vi "test_libssh2_channel_get_exit_signal.vi"() -> ()   [LabVIEW 2017, in "integration_tests.lvlib"]
uses:
  integration_tests.lvlib
  libssh2/libssh2_channel_open_ex.vi
  libssh2/libssh2_channel_process_startup.vi
  support/support.lvlib
  libssh2/libssh2.lvlib
  <vilib>/PNR/Transparent Assertions/Transparent Assertions/Transparent Assertions.lvlib
panel:
  out "error out":errorcluster
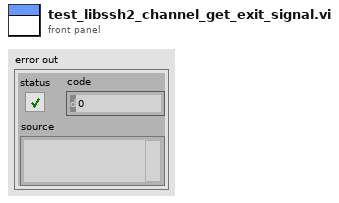
[diagram p1: front panel]
types:
  T1 = typedef "libssh2.lvlib/Session Refnum.ctl" = refnum<k1>
  T2 = typedef "libssh2.lvlib/Channel Refnum.ctl" = refnum<k1>
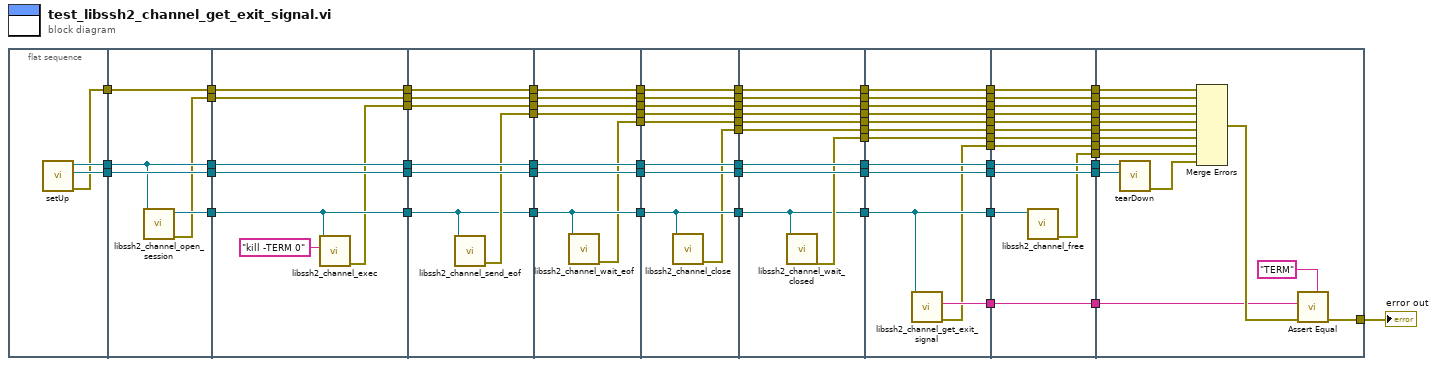
[diagram p0: block diagram]
diagram:
  n1 = flat-sequence {
    tunnel: [w76] -> w73
    tunnel: [w75] -> w72
    tunnel: [w74] -> w71
    tunnel: w73 -> [w80]
    tunnel: w72 -> [w81]
    tunnel: [w80] -> w70
    tunnel: [w81] -> w69
    tunnel: [w79] -> w68
    tunnel: w71 -> [w78]
    tunnel: [w78] -> w67
    tunnel: [w77] -> w66
    tunnel: w70 -> [w88]
    tunnel: [w88] -> w65
    tunnel: w69 -> [w87]
    tunnel: [w87] -> w64
    tunnel: w68 -> [w84]
    tunnel: [w84] -> w63
    tunnel: w67 -> [w86]
    tunnel: [w86] -> w62
    tunnel: w66 -> [w83]
    tunnel: [w83] -> w61
    tunnel: [w82] -> w60
    tunnel: w65 -> [w95]
    tunnel: [w95] -> w19
    tunnel: w64 -> [w94]
    tunnel: [w94] -> w17
    tunnel: w63 -> [w89]
    tunnel: [w89] -> w15
    tunnel: w62 -> [w93]
    tunnel: [w93] -> w13
    tunnel: w61 -> [w92]
    tunnel: [w92] -> w11
    tunnel: w60 -> [w91]
    tunnel: [w91] -> w9
    tunnel: [w90] -> w7
    tunnel: w19 -> [w103]
    tunnel: [w103] -> w18
    tunnel: w17 -> [w102]
    tunnel: [w102] -> w16
    tunnel: w15 -> [w97]
    tunnel: [w97] -> w14
    tunnel: w13 -> [w101]
    tunnel: [w101] -> w12
    tunnel: w11 -> [w100]
    tunnel: [w100] -> w10
    tunnel: w9 -> [w99]
    tunnel: [w99] -> w8
    tunnel: w7 -> [w98]
    tunnel: [w98] -> w6
    tunnel: [w96] -> w5
    tunnel: w18 -> [w112]
    tunnel: w16 -> [w111]
    tunnel: w14 -> [w110]
    tunnel: [w112] -> w38
    tunnel: [w111] -> w36
    tunnel: [w110] -> w34
    tunnel: [w109] -> w32
    tunnel: w12 -> [w108]
    tunnel: [w108] -> w30
    tunnel: w10 -> [w107]
    tunnel: [w107] -> w28
    tunnel: w8 -> [w106]
    tunnel: [w106] -> w26
    tunnel: w6 -> [w105]
    tunnel: [w105] -> w24
    tunnel: w5 -> [w104]
    tunnel: [w104] -> w4
    tunnel: w38 -> [w122]
    tunnel: [w122] -> w37
    tunnel: w36 -> [w121]
    tunnel: [w121] -> w35
    tunnel: w34 -> [w114]
    tunnel: [w114] -> w33
    tunnel: w32 -> [w120]
    tunnel: [w120] -> w31
    tunnel: w30 -> [w119]
    tunnel: [w119] -> w29
    tunnel: w28 -> [w118]
    tunnel: [w118] -> w27
    tunnel: w26 -> [w117]
    tunnel: [w117] -> w25
    tunnel: w24 -> [w116]
    tunnel: [w116] -> w23
    tunnel: [w115] -> w22
    tunnel: w4 -> [w113]
    tunnel: [w113] -> w3
    tunnel: w37 -> [w134]
    tunnel: [w134] -> w50
    tunnel: w35 -> [w133]
    tunnel: [w133] -> w49
    tunnel: w33 -> [w126]
    tunnel: [w126] -> w48
    tunnel: w31 -> [w132]
    tunnel: [w132] -> w47
    tunnel: w29 -> [w131]
    tunnel: [w131] -> w46
    tunnel: w27 -> [w130]
    tunnel: [w130] -> w45
    tunnel: w25 -> [w129]
    tunnel: [w129] -> w44
    tunnel: w23 -> [w128]
    tunnel: [w128] -> w43
    tunnel: [w127] -> w41
    tunnel: [w125] -> w40
    tunnel: w22 -> [w124]
    tunnel: [w124] -> w21
    tunnel: w3 -> [w123]
    tunnel: [w123] -> w2
    tunnel: w50 -> [w147]
    tunnel: w49 -> [w146]
    tunnel: w48 -> [w145]
    tunnel: [w147] -> w59
    tunnel: [w146] -> w58
    tunnel: [w144] -> w57
    tunnel: w47 -> [w143]
    tunnel: [w143] -> w56
    tunnel: w46 -> [w142]
    tunnel: [w142] -> w55
    tunnel: w45 -> [w141]
    tunnel: [w141] -> w54
    tunnel: w44 -> [w140]
    tunnel: [w140] -> w53
    tunnel: w43 -> [w139]
    tunnel: [w139] -> w52
    tunnel: [w138] -> w42
    tunnel: w41 -> [w138]
    tunnel: w40 -> [w137]
    tunnel: [w137] -> w39
    tunnel: w21 -> [w136]
    tunnel: [w136] -> w20
    tunnel: w2 -> [w135]
    tunnel: [w135] -> w1
    tunnel: w59 -> [w163]
    tunnel: w58 -> [w162]
    tunnel: [w161] -> w51
    tunnel: w57 -> [w159]
    tunnel: w56 -> [w158]
    tunnel: w55 -> [w157]
    tunnel: w54 -> [w155]
    tunnel: w53 -> [w154]
    tunnel: w52 -> [w153]
    tunnel: w42 -> [w152]
    tunnel: w39 -> [w151]
    tunnel: w20 -> [w149]
    tunnel: w1 -> [w148]
    frame #0 {
      n2 = call "setUp.vi"() -> ("error out"=w74:errorcluster, "connection ID"=w75:refnum<k5>, "session"=w76:T1)  [unwired: 9 in]
    }
    frame #1 {
      n3 = call "libssh2_channel_open_session.vi"("session"=w80) -> ("error out"=w77:errorcluster, "channel"=w79:T2)  [unwired: 9 in]
    }
    frame #2 {
      n4 = call "libssh2_channel_exec.vi"("command"="kill -TERM 0", "channel"=w84) -> ("error out"=w82:errorcluster)  [unwired: 9 in]
    }
    frame #3 {
      n5 = call "libssh2_channel_send_eof.vi"("channel"=w89) -> ("error out"=w90:errorcluster)  [unwired: 10 in]
    }
    frame #4 {
      n6 = call "libssh2_channel_wait_eof.vi"("channel"=w97) -> ("error out"=w96:errorcluster)  [unwired: 10 in]
    }
    frame #5 {
      n7 = call "libssh2_channel_close.vi"("channel"=w110) -> ("error out"=w109:errorcluster)  [unwired: 10 in]
    }
    frame #6 {
      n8 = call "libssh2_channel_wait_closed.vi"("channel"=w114) -> ("error out"=w115:errorcluster)  [unwired: 10 in]
    }
    frame #7 {
      n9 = call "libssh2_channel_get_exit_signal.vi"("channel"=w126) -> ("error out"=w125:errorcluster, "exitsignal"=w127:string)  [unwired: 7 in, 2 out]
    }
    frame #8 {
      n10 = call "libssh2_channel_free.vi"("channel"=w145) -> ("error out"=w144:errorcluster)  [unwired: 10 in]
    }
    frame #9 {
      n11 = call "tearDown.vi"("connection ID"=w162, "session"=w163) -> ("error out"=w160:errorcluster)  [unwired: 9 in]
      n12 = Merge Errors(w157, w155, w154, w153, w148, w158, w149, w151, w159, w160) -> (w156:errorcluster)
      n13 = call <vilib>:"Assert Equal.vi"("Expected"="TERM" ("exitsignal"), "error in (no error)"=w156, "Actual"=w152) -> ("error out"=w161:errorcluster)  [unwired: 8 in]
    }
  }
  "error out" <- w51
